vi "direction_to_rotation.vi"(8 "To":dbl[](array[numeric]), 11 "From":dbl[](array[numeric])) -> (2 "Rotation":T1=[[1.0, 0.0, 0.0], [0.0, 1.0, 0.0], [0.0, 0.0, 1.0]])   [LabVIEW 2013]
uses:
  <vilib>/Analysis/Matrix/Datatypes/RealMatrix.ctl
  <vilib>/Analysis/baseanly.llb/A x Vector.vi
  norm_vec.vi
  magnitude_dbl.vi
  <vilib>/Analysis/NI_AALBase.lvlib
  <vilib>/Analysis/Matrix/NI_Matrix.lvlib
panel:
  # "Create a rotation matrix from two direction vectors (need not be normalized). The rotation maps the \"from\" vector onto the \"to\" vector, defining the unspecified rotation component so that there is no component of rotation about the \"from\" axis.  This is useful for pointing in a direction when we don't care about rotation around the axis (or we want it to be zero.)"
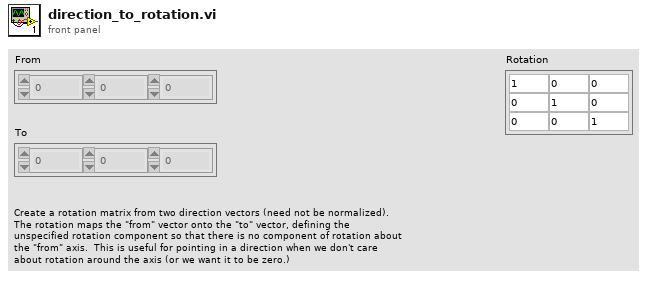
[diagram p1: front panel]
types:
  T1 = typedef "NI_Matrix.lvlib/RealMatrix.ctl" = dbl[][]
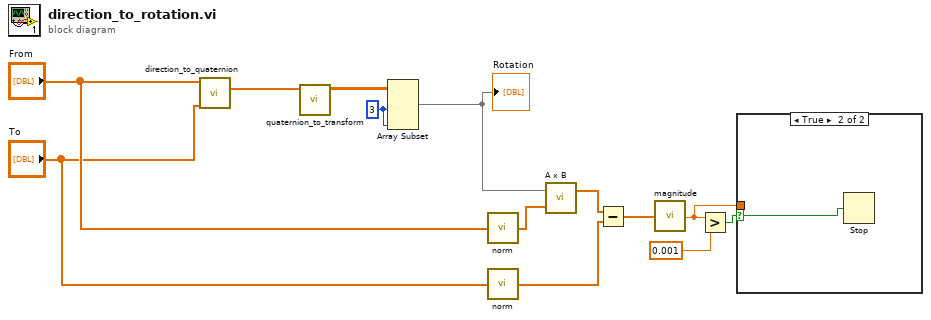
[diagram p0: block diagram]
diagram:
  w2 = 3 ("length")
  n1 = call "direction_to_quaternion.vi"("To"="To", "From"="From") -> ("Quaternion"=w4:dbl[])  [unwired: 9 in]
  n2 = call "quaternion_to_transform.vi"("Quaternion"=w4) -> ("Transform matrix"=w3:T1)  [unwired: 10 in]
  n3 = Array Subset(array=w3, length (row)=w2, length (col)=w2) -> (w1:T1)  [unwired: 2 in]
  "Rotation" <- w1
  n4 = call-poly "norm.vi"("vector"="From") -> ("normalized vector"=w13:dbl[])  [unwired: 3 in, 1 out]
  n5 = call-poly "norm.vi"("vector"="To") -> ("normalized vector"=w11:dbl[])  [unwired: 3 in, 1 out]
  n6 = call-poly <vilib>:"A x B.vi"("Vector"=w13, "A"=w1) -> ("A x Vector"=w12:dbl[])  [unwired: 1 out]
  n7 = Subtract(x=w12, y=w11) -> (x-y=w10:dbl[])
  n8 = call-poly "magnitude.vi"("vector"=w10) -> ("vector magnitude"=w7:dbl)  [unwired: 4 in]
  n9 = Greater?(x=w7, y=0.001) -> (0:w8:bool)
  n10 = case shown="True" w8 {
    selector: w8 -> [_ w14]
    tunnel: w7 -> [_ _]
    frame False {
    }
    frame True {
      n11 = Stop(stop? (T)=w14) -> ()
    }
  }
